vi "Test Master.vi"() -> ()   [LabVIEW 2024, in "Magnet module.lvlib"]
uses:
  Magnet module.lvlib
  ctl/SetField data.ctl
  ctl/Magnet mode.ctl
  <instrlib>/SMS drivers/Public/PSU Status.ctl
  <instrlib>/SMS drivers/Cryogenic Ltd SMSXXX.lvlib
  Messenger service/MessengerLib.lvlib
  ctl/MagnetStates.ctl
  ctl/MSG to magnet.ctl
  ctl/SetField.ctl
  ctl/Magnet config constants.ctl
  ctl/TM Revision.ctl
  ctl/Cryostat temperature sensors.ctl
  ctl/RampingOutput.ctl
  ctl/Overall status.ctl
  ctl/Change operation mode.ctl
  ctl/Magnet mode public.ctl
  ctl/Actual magnet state.ctl
  ctl/Magnet Orders.ctl
  Multi-HFEPR app/Datatypes/Connected modules.ctl
  Multi-HFEPR app/Datatypes/Magnet indicators.ctl
panel:
  in  "Polarity":bool=TRUE
  out "Array out":string[](array[string])
  in  "Magnet Config Constants":T1={"Switch resistant [K]"=5.0, "Switch superconducting [K]"=4.0, "First stage critical temperature [K]"=50.0, "Second stage critical temperature [K]"=5.0, "Inner magnet critical temperature [K]"=6.0, "Outer magnet critical temperature [K]"=5.0, "Field Constant [T/A]"=0.14911, "Maximum Current [A]"=107.3, "Maximum field [T]"=16.0, "Maximum source ramp [A/s]"=0.5, "Source precision [T]"=2e-05, "Ramp limits [A/s]"=[0.0506, 0.038, 0.0285, 0.0213, 0.0104], "Field limits [T]"=[3.0, 9.6, 13.3, 15.5, 16.0], "SMS"="COM3", "LSC218"="COM1"}
  in  "Stop Button":bool
  in  "Equalize":bool caption="Run State 2"
  in  "Zero":bool caption="Run State 2"
  in  "Start ramping":bool caption="Run State 2"
  in  "Magnet controls":T2
  out "Conversion\nconstant[T/A]":dbl
  out "Maximum field [T]":dbl
  out "SMS":refnum<visa-resource-name>
  out "LSC218":refnum<visa-resource-name>
  out "PSU Output [T]":dbl(slide) scale=0.0..16.0
  out "Magnet\nmodule\nupdated":bool=TRUE
  out "Field [T]":dbl(slide) scale=0.0..16.0
  out "Magnet indicators":T3={"Coil\noverheat"=FALSE, "Cryo-head\noverheat"=FALSE, "Switch T [K]"=0.0, "Actual field[T]"=0.0, "Heater"=FALSE, "Target\nreached"=FALSE, "Ramp[mT/s]"=0.0, "T monitor"="", "PSU"="", "Ramp limits[T/s]"=[], "Conversion\nconstant[T/A]"=0.0, "Last update"=0.0, "Field limits[T]"=[], "Voltage [V]"=16.0}
  out "Instruments status":T4
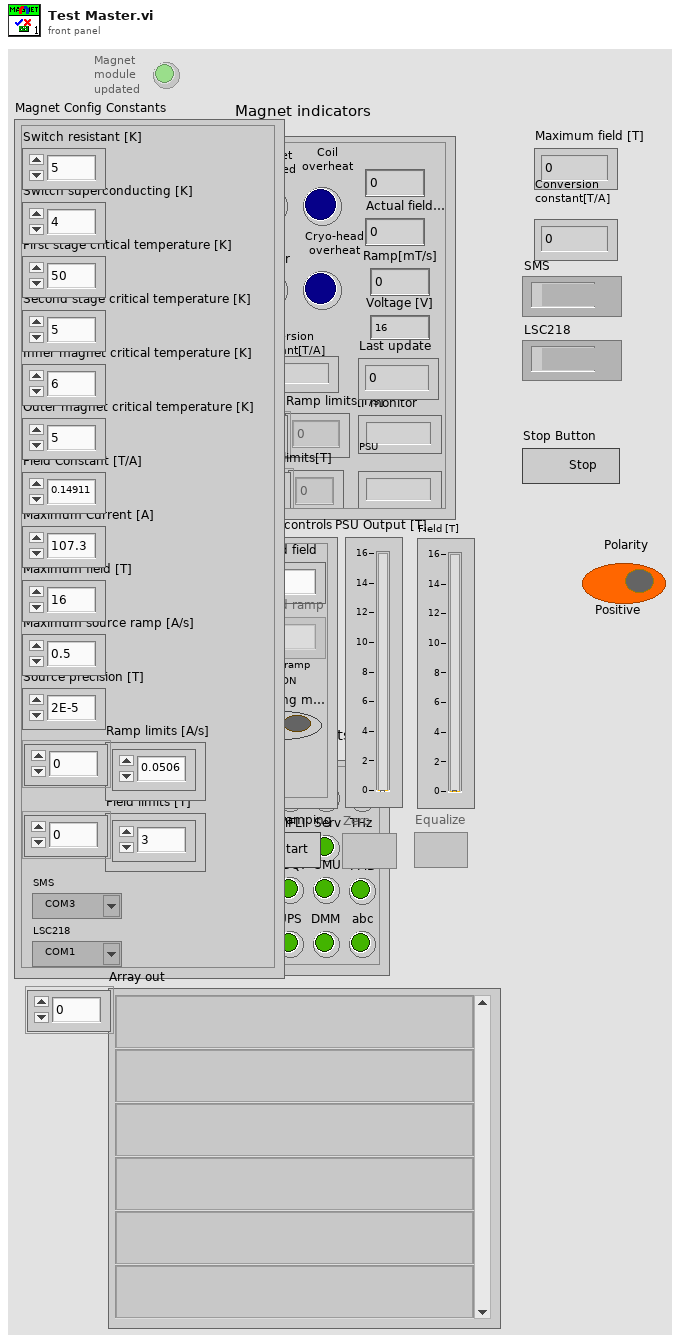
[diagram p1: front panel]
types:
  T1 = typedef "Magnet module.lvlib/Magnet config constants.ctl" = cluster{"Switch resistant [K]":dbl, "Switch superconducting [K]":dbl, "First stage critical temperature [K]":dbl, "Second stage critical temperature [K]":dbl, "Inner magnet critical temperature [K]":dbl, "Outer magnet critical temperature [K]":dbl, "Field Constant [T/A]":dbl, "Maximum Current [A]":dbl, "Maximum field [T]":dbl, "Maximum source ramp [A/s]":dbl, "Source precision [T]":dbl, "Ramp limits [A/s]":dbl[], "Field limits [T]":dbl[], "SMS":refnum<visa-resource-name>, "LSC218":refnum<visa-resource-name>}
  T2 = cluster{"Desired field":dbl, "Desired ramp":dbl, "Custom ramp":bool, "Ramping mode":bool}
  T3 = typedef "Magnet indicators.ctl" = cluster{"Coil\noverheat":bool, "Cryo-head\noverheat":bool, "Switch T [K]":dbl, "Actual field[T]":dbl, "Heater":bool, "Target\nreached":bool, "Ramp[mT/s]":dbl, "T monitor":string, "PSU":string, "Ramp limits[T/s]":dbl[], "Conversion\nconstant[T/A]":dbl, "Last update":dbl, "Field limits[T]":dbl[], "Voltage [V]":dbl}
  T4 = typedef "Connected modules.ctl" = cluster{"Mag":bool, "Rot":bool, "VTI":bool, "MFLI":bool, "Serv":bool, "THz":bool, "ADQ7":bool, "SMU":bool, "PMD":bool, "UPS":bool, "DMM":bool, "abc":bool}
  T5 = typedef "Magnet module.lvlib/MagnetStates.ctl" = enum16{"Initialize", "Regular check", "Check message", "Set Field", "Switch mode", "Restart", "Stop"}
  T6 = typedef "MessengerLib.lvlib/Messenger referencies.ctl" = cluster{"TOP":refnum<queue>, "Instr_M":refnum<queue>, "Field_C":refnum<queue>, "Tmp_M":refnum<queue>, "Tmp_C":refnum<queue>, "Table_C":refnum<queue>, "MW_C":refnum<queue>, "Data_Aq":refnum<queue>, "Mod_M":refnum<queue>, "Field_M":refnum<queue>, "Pwr_M":refnum<queue>, "Angle_C":refnum<queue>, "Sample_C":refnum<queue>, "Reserved":refnum<queue>}
  T7 = typedef "Magnet module.lvlib/MSG to magnet.ctl" = cluster{"Order":T8, "Data":variant}
  T8 = typedef "Magnet module.lvlib/Magnet Orders.ctl" = enum16{"Ignore", "Initialize", "Update", "Switch mode", "Set field", "Stop ramping", "Equalize output", "Zero output", "Flip polarity", "Blackout", "Disconnect", "End"}
  T9 = enum8{"Enabled", "Disabled", "Disabled and Grayed Out"}
  T10 = typedef "Magnet module.lvlib/MSG to magnet.ctl" = cluster{"Order":T11, "Data":variant}
  T11 = typedef "Magnet module.lvlib/Magnet Orders.ctl" = enum16{"Ignore", "Connect", "Update", "Switch mode", "Set field", "Stop ramping", "Equalize output", "Zero output", "Flip polarity", "Blackout", "Set timer", "Eval temperatures", "Disconnect"}
  T12 = typedef "Magnet module.lvlib/Change operation mode.ctl" = enum16{"Ramping", "Perzistant"}
  T13 = typedef "Magnet module.lvlib/SetField data.ctl" = cluster{"Field [T]":dbl, "Ramp [T/s]":dbl, "Custom Ramp?":bool, "Mode":T14}
  T14 = typedef "Magnet module.lvlib/Magnet mode public.ctl" = enum16{"Persistant", "Ramping"}
  T15 = typedef "Magnet module.lvlib/Cryostat temperature sensors.ctl" = cluster{"First stage A [K]":dbl, "Second stage A [K]":dbl, "Firs stage B [K]":dbl, "Second stage B [K]":dbl, "Inner magnet [K]":dbl, "Outer Magnet [K]":dbl, "Switch [K]":dbl, "Support plate [K]":dbl, "Time stamp":dbl}
  T16 = typedef "Magnet module.lvlib/RampingOutput.ctl" = enum16{"At Target", "Go up", "Go down"}
  T17 = typedef "Magnet module.lvlib/Magnet mode.ctl" = enum16{"Persistant", "Switching", "Ramping", "Quenched"}
  T18 = typedef "Magnet module.lvlib/Overall status.ctl" = cluster{"Desired":T13, "Actual":T19}
  T19 = typedef "Magnet module.lvlib/Actual magnet state.ctl" = cluster{"Mode":T17, "Ramping output":T16, "Ready for change":bool, "Switch heater":bool, "Cooler Overheat":bool, "Coil overheat":bool, "Energized":bool, "Output [T]":dbl, "Field [T]":dbl, "Ramp[T/s]":dbl, "Switch\ntemperature [K]":dbl, "Voltage [V]":dbl, "Current direction":bool}
  T20 = typedef "Magnet module.lvlib/SetField.ctl" = cluster{"Field[T]":dbl, "Ramp[T/s]":dbl, "Custom\nramp?":bool}
  T21 = typedef "Cryogenic Ltd SMSXXX.lvlib/PSU Status.ctl" = cluster{"Ramp Target":enum16{"ZERO", "MID", "MAX"}, "Pause":bool, "Switch Heater":bool, "Persistent Field":dbl, "Persistent Current":dbl, "Tesla":bool, "Output (T)":dbl, "Output (A)":dbl, "X Trip":enum16{"DISABLED", "ENABLED", "ACTIVE"}, "Ramp Rate (A/s)":dbl, "V Limit (V)":dbl, "Heater Voltage":dbl, "MAX Setpoint (A)":dbl, "MAX Setpoint (T)":dbl, "MID Setpoint (A)":dbl, "MID Setpoint (T)":dbl, "Lock":bool, "Field Constant":dbl, "Remote":bool, "Direction":enum16{"POSITIVE", "NEGATIVE", "OPEN", "UNIPOLAR"}, "Helium Level":u16, "Quench !":bool, "Voltage":dbl, "V Limit !":bool, "Ramping":bool, "At Target":bool, "Trip Field":dbl, "Trip Current":dbl}
  T22 = typedef "Magnet module.lvlib/TM Revision.ctl" = cluster{"Instr Serial Number":string, "Instr Driver Revision":string, "Instr Firmware Revision":string, "Instr Model Number":string}
  T23 = typedef "MessengerLib.lvlib/MSG to TOP.ctl" = cluster{"Module":T24, "Response":string, "Data":variant, "Time":timestamp}
  T24 = typedef "Module name.ctl" = enum16{"Emty", "Magnet", "VTI", "Excitation", "Servo", "Acquisition", "Rotator", "Digitizer", "SMU2450", "Carousel", "Multimeter", "Tmp monitor", "Power monitor"}
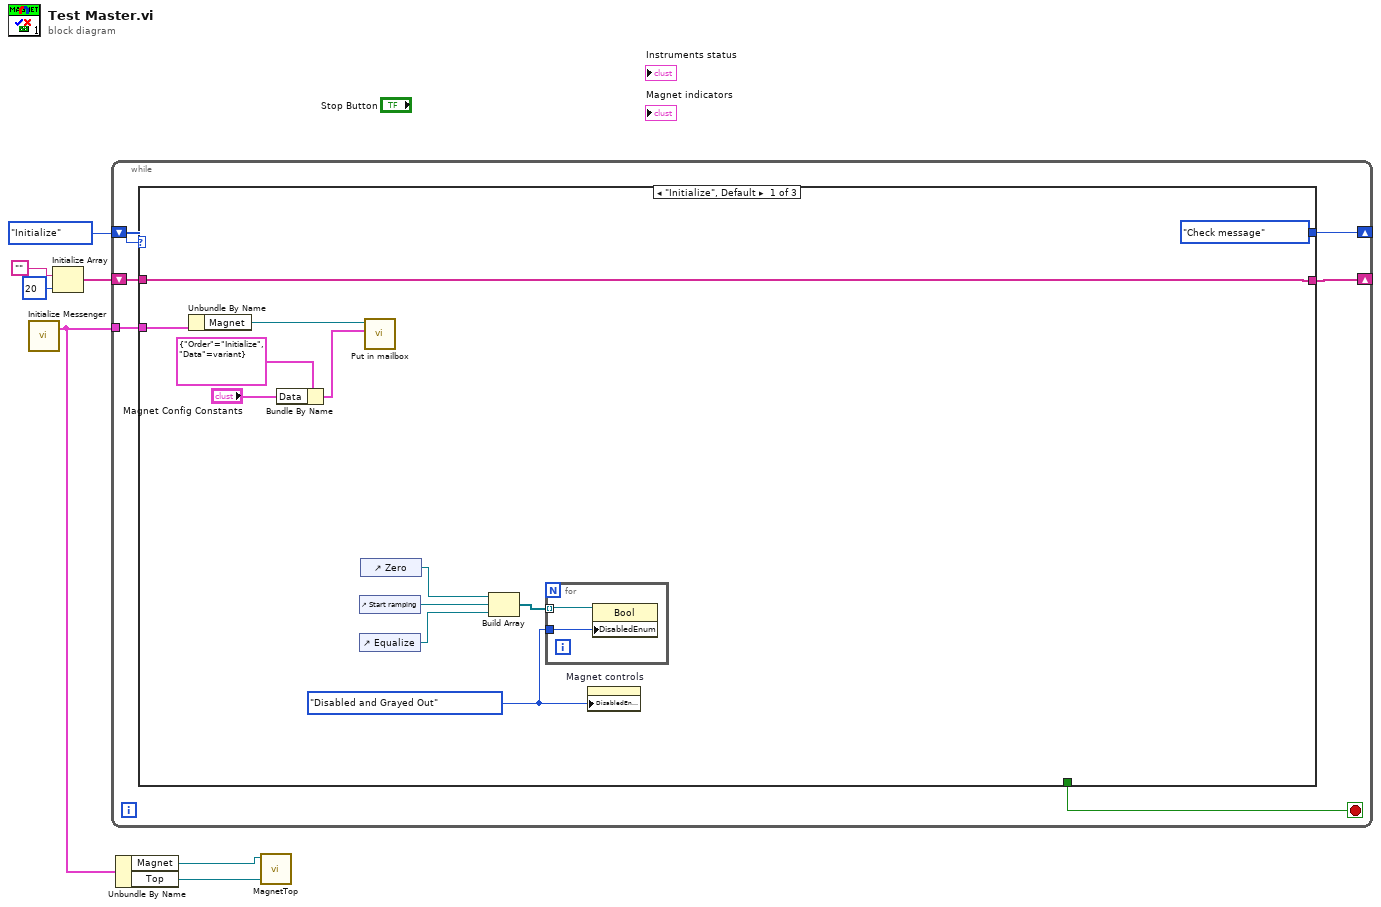
[diagram p0: block diagram]
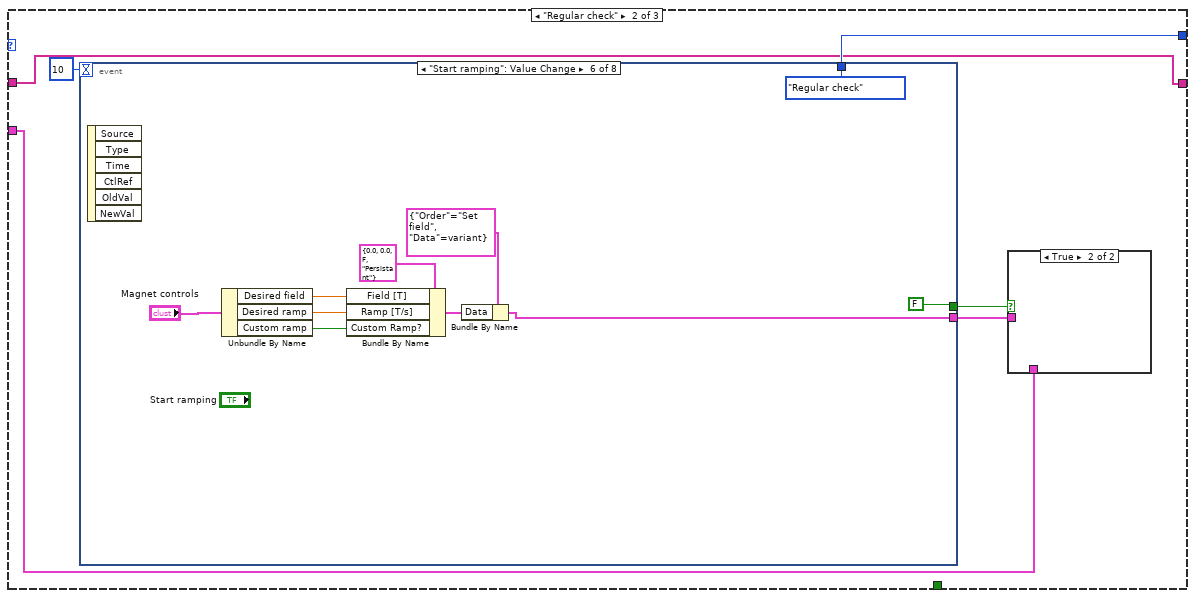
[diagram p2: hidden frame]
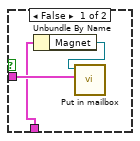
[diagram p3: hidden frame]
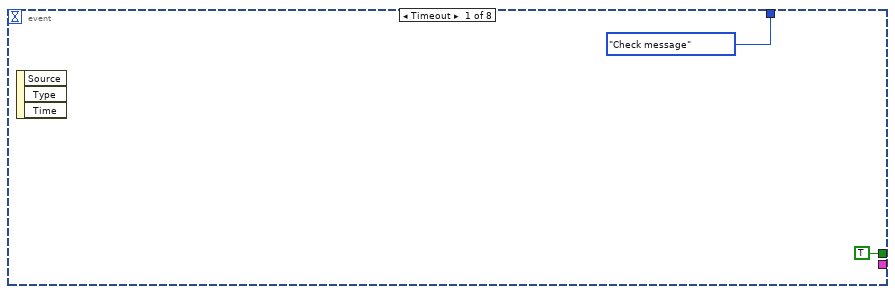
[diagram p4: hidden frame]
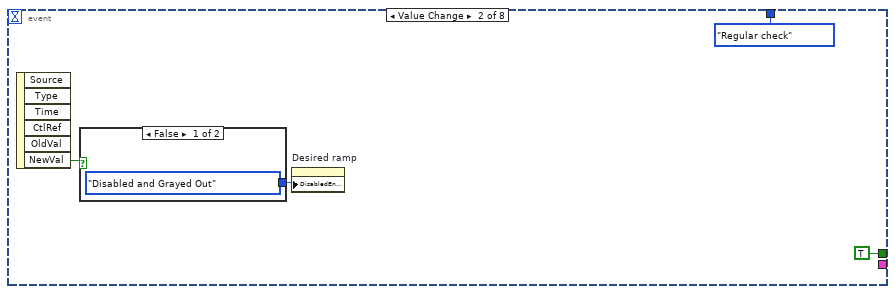
[diagram p5: hidden frame]
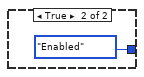
[diagram p6: hidden frame]
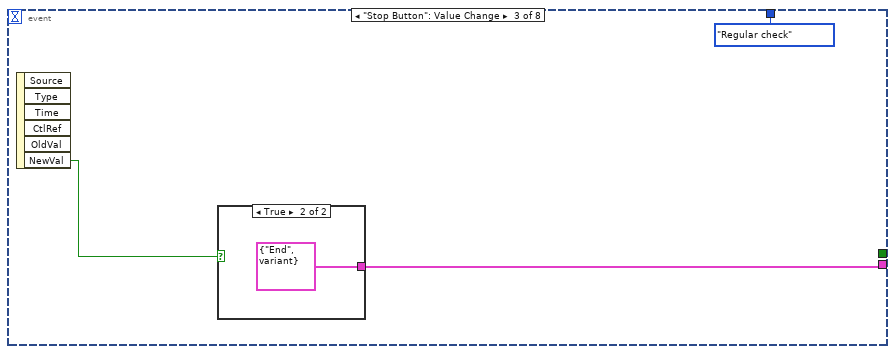
[diagram p7: hidden frame]
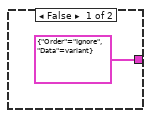
[diagram p8: hidden frame]
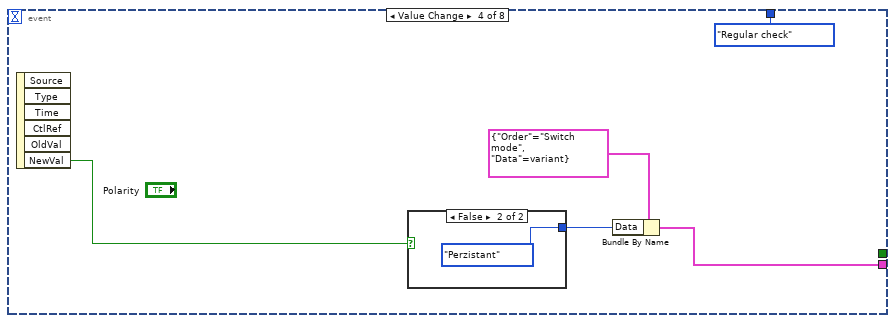
[diagram p9: hidden frame]
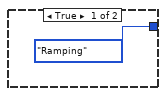
[diagram p10: hidden frame]
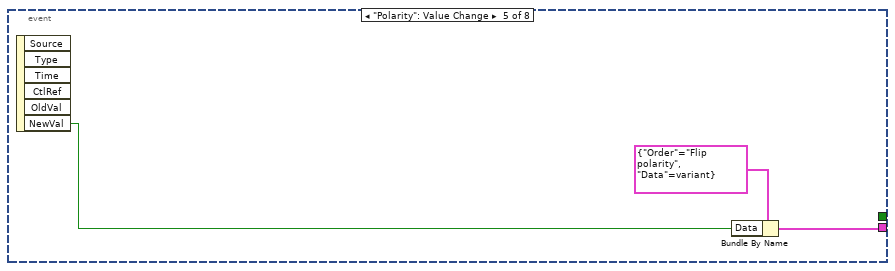
[diagram p11: hidden frame]
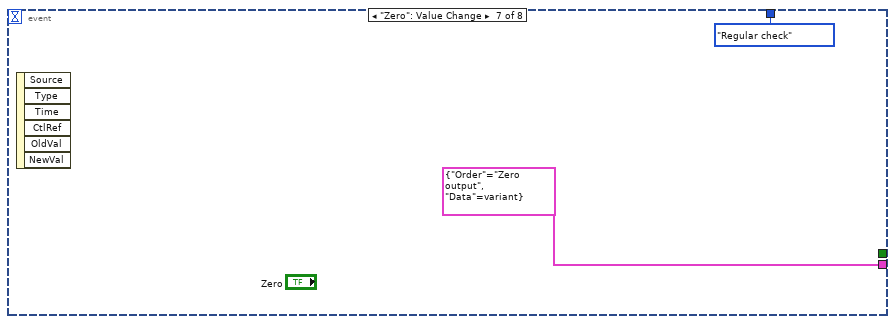
[diagram p12: hidden frame]
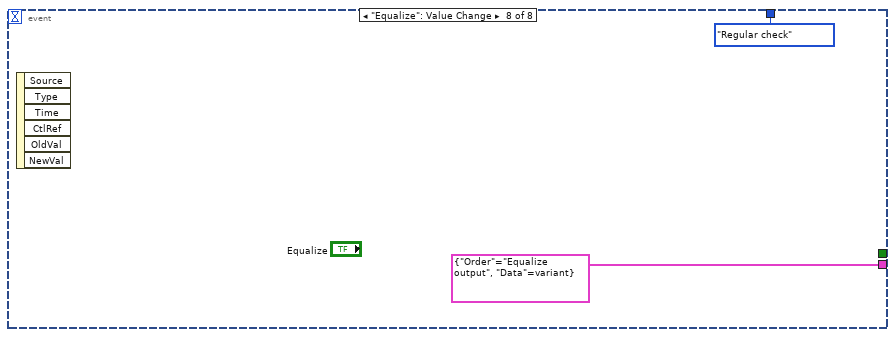
[diagram p13: hidden frame]
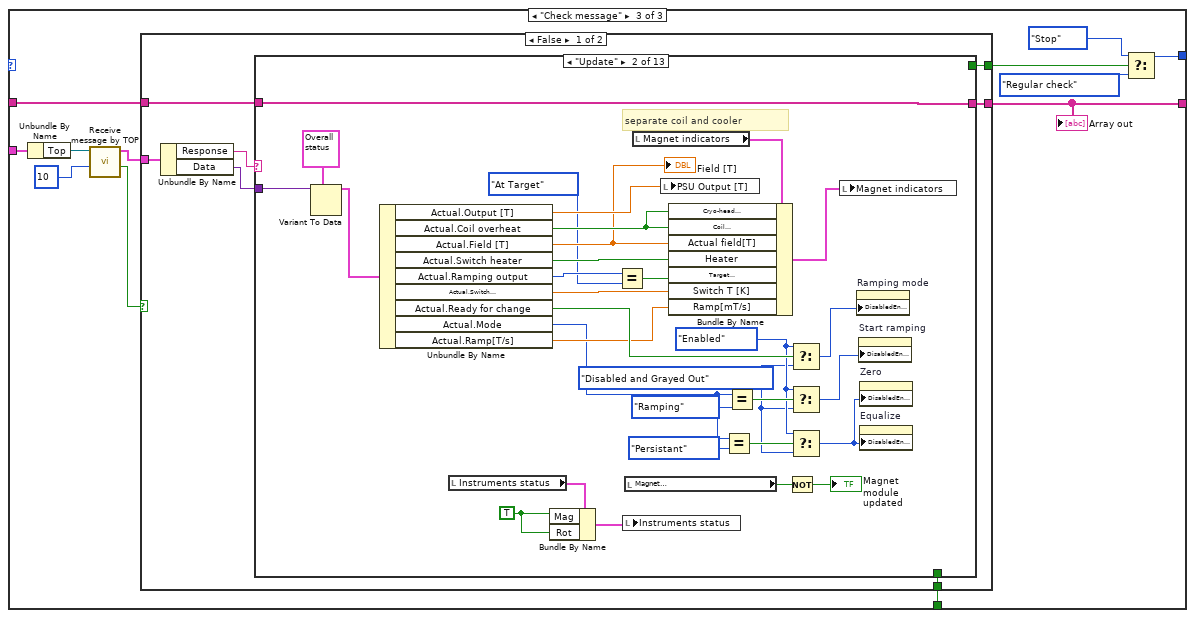
[diagram p14: hidden frame]
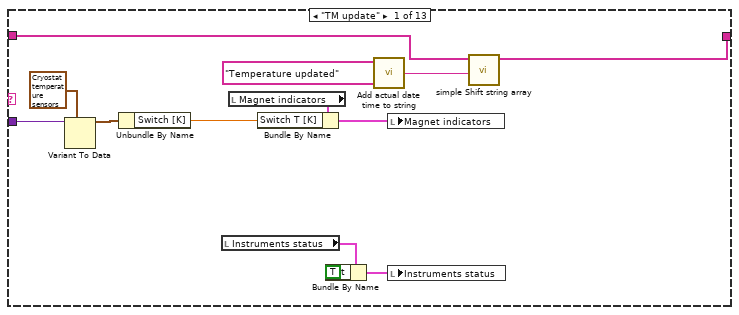
[diagram p15: hidden frame]
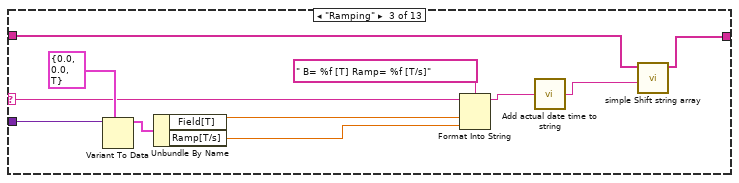
[diagram p16: hidden frame]
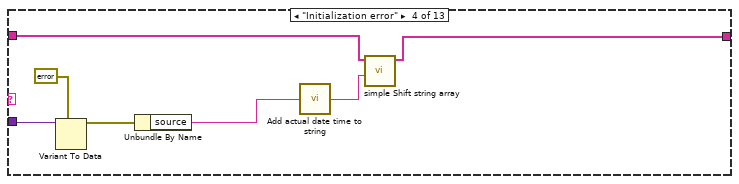
[diagram p17: hidden frame]
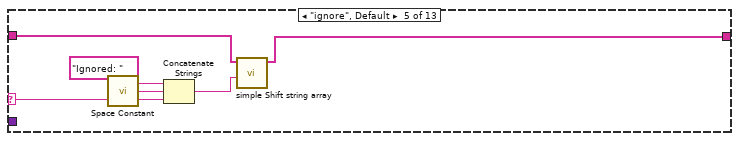
[diagram p18: hidden frame]
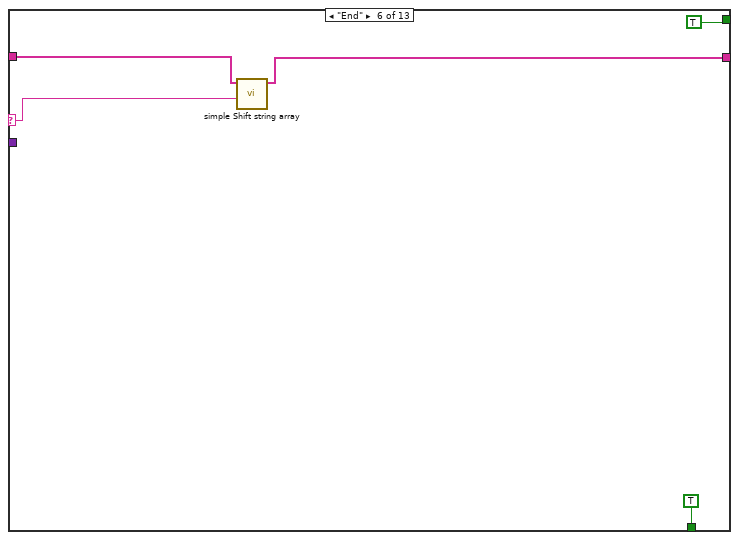
[diagram p19: hidden frame]
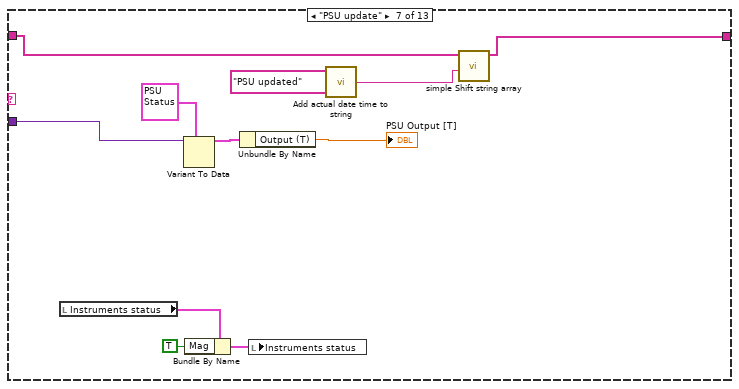
[diagram p20: hidden frame]
diagram:
  n1 = call "Initialize Messenger.vi"() -> ("Referencies out"=w3:T6)  [unwired: 2 in, 1 out]
  n2 = Initialize Array("", 20 ("dimension size")) -> (w5:string[])
  n3 = while {
    tunnel: w3 -> [w12]
    shift-right: [w10] -> _
    shift-left: w5 -> [w13]
    shift-right: [w9] -> _
    shift-left: MagnetStates."Initialize" ("State") -> [w11]
    stop <- w8 stop-if-true
    n4 = case shown="\"Initialize\", Default" w11 {
      tunnel: w13 -> [w15 w29 w82]
      tunnel: w12 -> [w19 w28 w81]
      tunnel: [w15 w29 w80] -> w10
      tunnel: [MagnetStates."Check message" ("State") w32 w78] -> w9
      tunnel: [_ _ w79] -> w8
      frame "Initialize", Default {
        w21 = T9."Disabled and Grayed Out" ("Disabled")
        n5 = Unbundle By Name(w19) -> ("Magnet"=w18:refnum<queue>)
        n6 = Bundle By Name(cluster=T7 {"Order"=enum."Initialize", "Data"=variant} ("MSG to magnet"), "Data"="Magnet Config Constants") -> (w17:T7)
        n7 = control-ref of="Start ramping"() -> (w25:refnum<vi>)
        n8 = control-ref of="Equalize"() -> (w24:refnum<vi>)
        n9 = control-ref of="Zero"() -> (w23:refnum<vi>)
        n10 = call "Put in mailbox.vi"("Message"=w17, "Queue in"=w18) -> ()  [unwired: 7 in, 3 out]
        n11 = Build Array(w23, w25, w24) -> (w22:refnum<vi>[])
        n12 = for {
          tunnel: w22 -> [w27] mode=indexing
          tunnel: w21 -> [w26]
          n13 = property class="Bool"(reference=w27, "DisabledEnum"=w26) -> ()  [unwired: 1 in, 2 out]
        }
        n14 = property on="Magnet controls" class="Clust (strict)"("DisabledEnum"=w21) -> ()  [unwired: 2 in, 2 out]
      }
      frame "Regular check" {
        n15 = event shown="[5] \"Start ramping\": Value Change" {
          selector: _ -> [_ _ _ _ _ _ _ _]
          dyn-events: _ -> [_ _ _ _ _ _ _ _]
          timeout: 10 -> [_ _ _ _ _ _ _ _]
          tunnel: [MagnetStates."Check message" ("State") MagnetStates."Regular check" ("State") MagnetStates."Regular check" ("State") MagnetStates."Regular check" ("State") _ MagnetStates."Regular check" ("State") MagnetStates."Regular check" ("State") MagnetStates."Regular check" ("State")] -> w32
          tunnel: [TRUE TRUE _ _ _ FALSE _ _] -> w31
          tunnel: [_ _ w46 w51 w59 w65 T10 {"Order"=enum."Zero output", "Data"=variant} ("MSG to magnet") T10 {"Order"=enum."Equalize output", "Data"=variant} ("MSG to magnet")] -> w30
          event Timeout {
            n16 = event-data() -> ()  [unwired: 1 in, 3 out]
          }
          event "Magnet controls.Custom ramp": Value Change {
            n17 = event-data() -> ("NewVal"=w42:bool)  [unwired: 1 in, 5 out]
            n18 = case shown="False" w42 {
              tunnel: [T9."Disabled and Grayed Out" ("Disabled") T9."Enabled" ("Disabled")] -> w41
              frame False {
              }
              frame True {
              }
            }
            n19 = property on="Desired ramp" class="DigNum (strict)"("DisabledEnum"=w41) -> ()  [unwired: 2 in, 2 out]
          }
          event "Stop Button": Value Change {
            n20 = event-data() -> ("NewVal"=w47:bool)  [unwired: 1 in, 5 out]
            n21 = case shown="True" w47 {
              tunnel: [T10 {"Order"=enum."Ignore", "Data"=variant} ("MSG to magnet") T7 {"Order"=enum."End", "Data"=variant} ("MSG to magnet")] -> w46
              frame False {
              }
              frame True {
              }
            }
          }
          event "Magnet controls.Ramping mode": Value Change {
            n22 = event-data() -> ("NewVal"=w53:bool)  [unwired: 1 in, 5 out]
            n23 = case shown="False" w53 {
              tunnel: [Change_operation_mode."Ramping" ("Operation mode") Change_operation_mode."Perzistant" ("Operation mode")] -> w52
              frame True {
              }
              frame False {
              }
            }
            n24 = Bundle By Name(cluster=T10 {"Order"=enum."Switch mode", "Data"=variant} ("MSG to magnet"), "Data"=w52) -> (w51:T10)
          }
          event "Polarity": Value Change {
            n25 = event-data() -> ("NewVal"=w57:bool)  [unwired: 1 in, 5 out]
            n26 = Bundle By Name(cluster=T10 {"Order"=enum."Flip polarity", "Data"=variant} ("MSG to magnet"), "Data"=w57) -> (w59:T10)
          }
          event "Start ramping": Value Change {
            n27 = event-data() -> ()  [unwired: 1 in, 6 out]
            n28 = Unbundle By Name("Magnet controls") -> ("Desired field"=w62:dbl, "Desired ramp"=w61:dbl, "Custom ramp"=w60:bool)
            n29 = Bundle By Name(cluster=T13 {"Field [T]"=0.0, "Ramp [T/s]"=0.0, "Custom Ramp?"=FALSE, "Mode"=enum."Persistant"} ("Set Field"), "Field [T]"=w62, "Ramp [T/s]"=w61, "Custom Ramp?"=w60) -> (w66:T13)
            n30 = Bundle By Name(cluster=T10 {"Order"=enum."Set field", "Data"=variant} ("MSG to magnet"), "Data"=w66) -> (w65:T10)
          }
          event "Zero": Value Change {
            n31 = event-data() -> ()  [unwired: 1 in, 6 out]
          }
          event "Equalize": Value Change {
            n32 = event-data() -> ()  [unwired: 1 in, 6 out]
          }
        }
        n33 = case shown="True" w31 {
          tunnel: w30 -> [w36 _]
          tunnel: w28 -> [w35 _]
          frame False {
            n34 = Unbundle By Name(w35) -> ("Magnet"=w34:refnum<queue>)
            n35 = call "Put in mailbox.vi"("Message"=w36, "Queue in"=w34) -> ()  [unwired: 7 in, 3 out]
          }
          frame True {
          }
        }
      }
      frame "Check message" {
        n36 = Unbundle By Name(w81) -> ("Top"=w85:refnum<queue>)
        n37 = call "Receive message by TOP.vi"("timeout (100)"=10 ("timeout in ms (-1)"), "Mailbox in"=w85) -> ("timed out?"=w74:bool, "MSG packet"=w84:T23)  [unwired: 6 in, 2 out]
        n38 = case shown="False" w74 {
          tunnel: w84 -> [w92 _]
          tunnel: w82 -> [w89 w263]
          tunnel: [w88 w263] -> w80
          tunnel: [w87 _] -> w79
          tunnel: [w86 _] -> w77
          frame False {
            n39 = Unbundle By Name(w92) -> ("Response"=w91:string, "Data"=w90:variant)
            n40 = case shown="\"Update\"" w91 {
              selector: w91 -> [_ _ w143 _ w159 w163 _ _ _ _ _ w247 _]
              tunnel: w90 -> [w97 w136 w147 w154 _ _ w173 w197 w206 w223 w239 w249 w262]
              tunnel: w89 -> [w93 w117 w138 w150 w156 w165 w166 w177 w200 w212 w226 w250 w253]
              tunnel: [w94 w117 w137 w149 w155 w164 w168 w178 w201 w213 w225 w251 w254] -> w88
              tunnel: [_ _ _ _ _ TRUE _ _ _ _ _ _ _] -> w87
              tunnel: [_ _ _ _ _ TRUE _ _ _ _ _ _ _] -> w86
              frame "TM update" {
                n41 = Variant To Data(type=T15 {"First stage A [K]"=0.0, "Second stage A [K]"=0.0, "Firs stage B [K]"=0.0, "Second stage B [K]"=0.0, "Inner magnet [K]"=0.0, "Outer Magnet [K]"=0.0, "Switch [K]"=0.0, "Support plate [K]"=0.0, "Time stamp"=0.0} ("LSC218 sensors"), Variant=w97) -> (data=w101:T15)  [unwired: 1 in, 1 out]
                n42 = Unbundle By Name(w101) -> ("Switch [K]"=w98:dbl)
                n43 = local read "Instruments status"() -> (w105:T4)
                n44 = local read "Magnet indicators"() -> (w99:T3)
                n45 = Bundle By Name(cluster=w99, "Switch T [K]"=w98) -> (w100:T3)
                n46 = Bundle By Name(cluster=w105, "Rot"=TRUE ("TM")) -> (w103:T4)
                n47 = call "Add actual date time to string.vi"("String in"="Temperature updated") -> ("String out"=w95:string)  [unwired: 4 in]
                n48 = local write "Magnet indicators"(w100) -> ()
                n49 = local write "Instruments status"(w103) -> ()
                n50 = call "simple Shift string array.vi"("Element in"=w95, "Array in"=w93) -> ("Array out"=w94:string[])  [unwired: 8 in, 1 out]
              }
              frame "Update" {
                w121 = TRUE ("PSU")
                w112 = T9."Disabled and Grayed Out" ("f")
                w116 = T9."Enabled" ("Disabled")
                # "separate coil and cooler"
                n51 = Variant To Data(type=T18 {"Desired"={"Field [T]"=0.0, "Ramp [T/s]"=0.0, "Custom Ramp?"=TRUE, "Mode"=enum."Ramping"}, "Actual"={"Mode"=enum."Persistant", "Ramping output"=enum."At Target", "Ready for change"=FALSE, "Switch heater"=FALSE, "Cooler Overheat"=FALSE, "Coil overheat"=FALSE, "Energized"=FALSE, "Output [T]"=0.0, "Field [T]"=0.0, "Ramp[T/s]"=0.0, "Switch\ntemperature [K]"=0.0, "Voltage [V]"=0.0, "Current direction"=FALSE}} ("output cluster"), Variant=w136) -> (data=w132:T18)  [unwired: 1 in, 1 out]
                n52 = Unbundle By Name(w132) -> ("Actual.Output [T]"=w124:dbl, "Actual.Coil overheat"=w130:bool, "Actual.Field [T]"=w111:dbl, "Actual.Switch heater"=w131:bool, "Actual.Ramping output"=w108:T16, "Actual.Switch\ntemperature [K]"=w125:dbl, "Actual.Ready for change"=w126:bool, "Actual.Mode"=w115:T17, "Actual.Ramp[T/s]"=w120:dbl)
                "Field [T]" <- w111
                n53 = local read "Instruments status"() -> (w123:T4)
                n54 = Bundle By Name(cluster=w123, "Mag"=w121, "Rot"=w121) -> (w122:T4)
                n55 = Equal?(x=w108, y=RampingOutput."At Target") -> (x = y?=w106:bool)
                n56 = local write "Instruments status"(w122) -> ()
                n57 = local read "Magnet\nmodule\nupdated"() -> (w119:bool)
                n58 = local read "Magnet indicators"() -> (w134:T3)
                n59 = local write "PSU Output [T]"(w124) -> ()
                n60 = Bundle By Name(cluster=w134, "Cryo-head\noverheat"=w130, "Coil\noverheat"=w130, "Actual field[T]"=w111, "Heater"=w131, "Target\nreached"=w106, "Switch T [K]"=w125, "Ramp[mT/s]"=w120) -> (w135:T3)
                n61 = Equal?(x=w115, y=Magnet_mode."Persistant") -> (x = y?=w113:bool)
                n62 = Equal?(x=w115, y=Magnet_mode."Ramping" ("Mode")) -> (x = y?=w128:bool)
                n63 = Not(x=w119) -> (.not. x?=→"Magnet\nmodule\nupdated":bool)
                n64 = Select(t=w116, s=w126, f=w112) -> (s? t:f=w129:T9)
                n65 = Select(t=w116, s=w128, f=w112) -> (s? t:f=w109:T9)
                n66 = Select(t=w116, s=w113, f=w112) -> (s? t:f=w110:T9)
                n67 = local write "Magnet indicators"(w135) -> ()
                n68 = property on="Ramping mode" class="Bool (strict)"("DisabledEnum"=w129) -> ()  [unwired: 2 in, 2 out]
                n69 = property on="Start ramping" class="Bool"("DisabledEnum"=w109) -> ()  [unwired: 2 in, 2 out]
                n70 = property on="Zero" class="Bool"("DisabledEnum"=w110) -> ()  [unwired: 2 in, 2 out]
                n71 = property on="Equalize" class="Bool"("DisabledEnum"=w110) -> ()  [unwired: 2 in, 2 out]
              }
              frame "Ramping" {
                n72 = Variant To Data(type=T20 {"Field[T]"=0.0, "Ramp[T/s]"=0.0, "Custom\nramp?"=TRUE} ("Set field"), Variant=w147) -> (data=w145:T20)  [unwired: 1 in, 1 out]
                n73 = Unbundle By Name(w145) -> ("Field[T]"=w142:dbl, "Ramp[T/s]"=w141:dbl)
                n74 = Format Into String(format string=" B= %f [T] Ramp= %f [T/s]", initial string=w143, w142, w141) -> (resulting string=w140:string)  [unwired: 1 in, 1 out]
                n75 = call "Add actual date time to string.vi"("String in"=w140) -> ("String out"=w139:string)  [unwired: 4 in]
                n76 = call "simple Shift string array.vi"("Element in"=w139, "Array in"=w138) -> ("Array out"=w137:string[])  [unwired: 8 in, 1 out]
              }
              frame "Initialization error" {
                n77 = Variant To Data(type=errorcluster {"status"=FALSE, "code"=0, "source"=""} ("error constant"), Variant=w154) -> (data=w152:errorcluster)  [unwired: 1 in, 1 out]
                n78 = Unbundle By Name(w152) -> ("source"=w151:string)
                n79 = call "Add actual date time to string.vi"("String in"=w151) -> ("String out"=w148:string)  [unwired: 4 in]
                n80 = call "simple Shift string array.vi"("Element in"=w148, "Array in"=w150) -> ("Array out"=w149:string[])  [unwired: 8 in, 1 out]
              }
              frame "ignore", Default {
                n81 = call <vilib>:"Space Constant.vi"() -> ("String"=w160:string)
                n82 = Concatenate Strings("Ignored: " ("String out"), w160, w159) -> (w157:string)
                n83 = call "simple Shift string array.vi"("Element in"=w157, "Array in"=w156) -> ("Array out"=w155:string[])  [unwired: 8 in, 1 out]
              }
              frame "End" {
                n84 = call "simple Shift string array.vi"("Element in"=w163, "Array in"=w165) -> ("Array out"=w164:string[])  [unwired: 8 in, 1 out]
              }
              frame "PSU update" {
                n85 = local read "Instruments status"() -> (w176:T4)
                n86 = Variant To Data(type=T21 {"Ramp Target"=enum."ZERO", "Pause"=FALSE, "Switch Heater"=FALSE, "Persistent Field"=0.0, "Persistent Current"=0.0, "Tesla"=FALSE, "Output (T)"=0.0, "Output (A)"=0.0, "X Trip"=enum."DISABLED", "Ramp Rate (A/s)"=0.0, "V Limit (V)"=0.0, "Heater Voltage"=0.0, "MAX Setpoint (A)"=0.0, "MAX Setpoint (T)"=0.0, "MID Setpoint (A)"=0.0, "MID Setpoint (T)"=0.0, "Lock"=FALSE, "Field Constant"=0.0, "Remote"=FALSE, "Direction"=enum."POSITIVE", "Helium Level"=0, "Quench !"=FALSE, "Voltage"=0.0, "V Limit !"=FALSE, "Ramping"=FALSE, "At Target"=FALSE, "Trip Field"=0.0, "Trip Current"=0.0} ("PSU Status Out"), Variant=w173) -> (data=w171:T21)  [unwired: 1 in, 1 out]
                n87 = Bundle By Name(cluster=w176, "Mag"=TRUE ("TM")) -> (w174:T4)
                n88 = Unbundle By Name(w171) -> ("Output (T)"=→"PSU Output [T]":dbl)
                n89 = local write "Instruments status"(w174) -> ()
                n90 = call "Add actual date time to string.vi"("String in"="PSU updated") -> ("String out"=w167:string)  [unwired: 4 in]
                n91 = call "simple Shift string array.vi"("Element in"=w167, "Array in"=w166) -> ("Array out"=w168:string[])  [unwired: 8 in, 1 out]
              }
              frame "Set field" {
                # "string for log"
                n92 = local read "Magnet controls"() -> (w195:T2)
                n93 = local read "Magnet indicators"() -> (w182:T3)
                n94 = Variant To Data(type=T13 {"Field [T]"=0.0, "Ramp [T/s]"=0.0, "Custom Ramp?"=TRUE, "Mode"=enum."Persistant"} ("Set Field"), Variant=w197) -> (data=w194:T13)  [unwired: 1 in, 1 out]
                n95 = Unbundle By Name(w194) -> ("Field [T]"=w187:dbl, "Ramp [T/s]"=w189:dbl, "Custom Ramp?"=w193:bool)
                n96 = Unbundle By Name(w195) -> ("Desired ramp"=w192:dbl)
                n97 = Unbundle By Name(w182) -> ("Actual field[T]"=w181:dbl)
                n98 = Not(x=w193) -> (.not. x?=w191:bool)
                n99 = call <userlib>:"MGI Approximately Equal.vi"("Numeric 2"=w192, "Numeric 1"=w189) -> ("approx = ?"=w190:bool)
                n100 = Or(x=w191, y=w190) -> (x .or. y?=w186:bool)
                n101 = case shown="False" w186 {
                  tunnel: ["Warning: Custom ramp was adjusted\n" ""] -> w184
                  frame False {
                  }
                  frame True {
                  }
                }
                n102 = Format Into String(format string="Setting magnetic field from %f [T ] to %f [T] with ramp %f [T/s]", w181, w187, w189) -> (resulting string=w185:string)  [unwired: 2 in, 1 out]
                n103 = Concatenate Strings(w185, "\r", w184) -> (w180:string)
                n104 = call "Add actual date time to string.vi"("String in"=w180) -> ("String out"=w179:string)  [unwired: 4 in]
                n105 = call "simple Shift string array.vi"("Element in"=w179, "Array in"=w177) -> ("Array out"=w178:string[])  [unwired: 8 in, 1 out]
              }
              frame "Switch mode" {
                n106 = Variant To Data(type=enum16{"Ramping", "Perzistant"}."Ramping" ("Operation mode"), Variant=w206) -> (data=w204:enum16{"Ramping", "Perzistant"})  [unwired: 1 in, 1 out]
                n107 = case shown="\"Perzistant\"" w204 {
                  tunnel: ["Switching to ramping mode" "Switching to perzistant mode"] -> w203
                  frame "Ramping", Default {
                  }
                  frame "Perzistant" {
                  }
                }
                n108 = call "Add actual date time to string.vi"("String in"=w203) -> ("String out"=w202:string)  [unwired: 4 in]
                n109 = call "simple Shift string array.vi"("Element in"=w202, "Array in"=w200) -> ("Array out"=w201:string[])  [unwired: 8 in, 1 out]
              }
              frame "Initialize" {
                w215 = TRUE ("PSU")
                w224 = T9."Enabled" ("Disabled")
                n110 = local read "Instruments status"() -> (w217:T4)
                n111 = Variant To Data(type="", Variant=w223) -> (data=w209:string)  [unwired: 1 in, 1 out]
                n112 = property on="Magnet controls" class="Clust (strict)"("DisabledEnum"=T9."Enabled" ("Disabled")) -> ()  [unwired: 2 in, 2 out]
                n113 = Unbundle By Name(T1 {"Switch resistant [K]"=5.0, "Switch superconducting [K]"=4.0, "First stage critical temperature [K]"=50.0, "Second stage critical temperature [K]"=5.0, "Inner magnet critical temperature [K]"=6.0, "Outer magnet critical temperature [K]"=5.0, "Field Constant [T/A]"=0.14911, "Maximum Current [A]"=107.3, "Maximum field [T]"=16.0, "Maximum source ramp [A/s]"=0.5, "Source precision [T]"=2e-05, "Ramp limits [A/s]"=[0.0506, 0.038, 0.0285, 0.0213, 0.0104], "Field limits [T]"=[3.0, 9.6, 13.3, 15.5, 16.0], "SMS"="", "LSC218"=""} ("Magnet Constants in")) -> ("Field Constant [T/A]"=→"Conversion\nconstant[T/A]":dbl, "Maximum field [T]"=→"Maximum field [T]":dbl, "SMS"=→"SMS":refnum<visa-resource-name>, "LSC218"=→"LSC218":refnum<visa-resource-name>)
                n114 = Bundle By Name(cluster=w217, "Mag"=w215, "Rot"=w215) -> (w216:T4)
                n115 = local write "Instruments status"(w216) -> ()
                n116 = property on="Rot" class="Bool (strict)"("DisabledEnum"=w224) -> ()  [unwired: 2 in, 2 out]
                n117 = property on="Mag" class="Bool (strict)"("DisabledEnum"=w224) -> ()  [unwired: 2 in, 2 out]
                n118 = call "Add actual date time to string.vi"("String in"=w209) -> ("String out"=w214:string)  [unwired: 4 in]
                n119 = call "simple Shift string array.vi"("Element in"=w214, "Array in"=w212) -> ("Array out"=w213:string[])  [unwired: 8 in, 1 out]
              }
              frame "Update error" {
                # "ReInitialize Magnet?"
                # "TODO: Logg error message"
                n120 = Variant To Data(type=errorcluster {"status"=FALSE, "code"=0, "source"=""} ("error in (no error)"), Variant=w239) -> (data=w236:errorcluster)  [unwired: 1 in, 1 out]
                n121 = Unbundle By Name(w236) -> ("source"=w233:string)
                n122 = Match Pattern(string=w233, regular expression="PSU") -> (offset past match=w231:i32)  [unwired: 1 in, 3 out]
                n123 = local read "Instruments status"() -> (w229:T4)
                n124 = Greater Than 0?(x=w231) -> (x > 0?=w230:bool)
                n125 = property on="Magnet controls" class="Clust (strict)"("DisabledEnum"=T9."Disabled and Grayed Out" ("Disabled")) -> ()  [unwired: 2 in, 2 out]
                n126 = case shown="True" w230 {
                  tunnel: w229 -> [w241 w244]
                  tunnel: [w242 w243] -> w228
                  frame False {
                    n127 = Bundle By Name(cluster=w241, "Rot"=FALSE ("TM")) -> (w242:T4)
                  }
                  frame True {
                    n128 = Bundle By Name(cluster=w244, "Mag"=FALSE ("PSU")) -> (w243:T4)
                  }
                }
                n129 = Concatenate Strings("Magnet Update error" ("String in"), w233) -> (w234:string)
                n130 = call "Add actual date time to string.vi"("String in"=w234) -> ("String out"=w227:string)  [unwired: 4 in]
                n131 = local write "Instruments status"(w228) -> ()
                n132 = call "simple Shift string array.vi"("Element in"=w227, "Array in"=w226) -> ("Array out"=w225:string[])  [unwired: 8 in, 1 out]
              }
              frame "Flip polarity" {
                n133 = Variant To Data(type=w247, Variant=w249) -> (data=w248:string)  [unwired: 1 in, 1 out]
                n134 = Concatenate Strings(w247, w248) -> (w246:string)
                n135 = call "Add actual date time to string.vi"("String in"=w246) -> ("String out"=w252:string)  [unwired: 4 in]
                n136 = call "simple Shift string array.vi"("Element in"=w252, "Array in"=w250) -> ("Array out"=w251:string[])  [unwired: 8 in, 1 out]
              }
              frame "TM revision" {
                # "TODO: Logg temperature monitor  message"
                n137 = Variant To Data(type=T22 {"Instr Serial Number"="", "Instr Driver Revision"="", "Instr Firmware Revision"="", "Instr Model Number"=""} ("TM Revision"), Variant=w262) -> (data=w260:T22)  [unwired: 1 in, 1 out]
                n138 = Unbundle By Name(w260) -> ("Instr Model Number"=w259:string)
                n139 = call <vilib>:"Space Constant.vi"() -> ("String"=w257:string)
                n140 = Concatenate Strings("Temperature monitor:" ("string"), w257, w259) -> (w256:string)
                n141 = call "Add actual date time to string.vi"("String in"=w256) -> ("String out"=w255:string)  [unwired: 4 in]
                n142 = call "simple Shift string array.vi"("Element in"=w255, "Array in"=w253) -> ("Array out"=w254:string[])  [unwired: 8 in, 1 out]
              }
            }
          }
          frame True {
          }
        }
        "Array out" <- w80
        n143 = Select(t=MagnetStates."Stop" ("f"), s=w77, f=MagnetStates."Regular check" ("State")) -> (s? t:f=w78:T5)
      }
    }
  }
  n144 = Unbundle By Name(w3) -> ("Magnet"=w2:refnum<queue>, "Top"=w1:refnum<queue>)
  n145 = call "MagnetTop.vi"("Queue to UI"=w1, "Module queue"=w2) -> ()  [unwired: 10 in]
